vi "INITIALIZE DB CONNECTION.vi"(8 "error in (no error)":errorcluster, 9 "Password":string, 10 "User Name":string="Admin", 11 "DB PATH":path=path "E:/LabView/PPLR DATABAS.udl") -> (0 "error out":errorcluster, 3 "CONNECTED?":bool)   [LabVIEW 2024]
uses:
  <vilib>/addons/database/Connection.llb/DB Tools Open Connec (Path).vi
  <vilib>/addons/database/NI_Database_API.lvlib
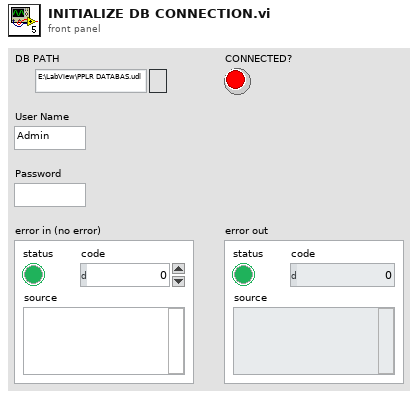
[diagram p1: front panel]
types:
  T1 = typedef "NI_Database_API.lvlib/Conn ObjectReference.ctl" = refnum<k1>
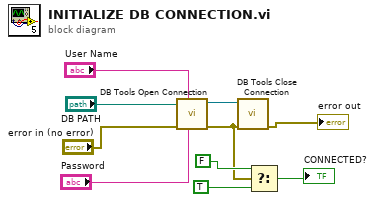
[diagram p0: block diagram]
diagram:
  n1 = call-poly <vilib>:"DB Tools Open Connection.vi"("password"="Password", "userID"="User Name", "error in (no error)"="error in (no error)", "connection information"="DB PATH") -> ("error out"=w7:errorcluster, "connection reference"=w5:T1)  [unwired: 4 in]
  n2 = call <vilib>:"DB Tools Close Connection.vi"("error in (no error)"=w7, "connection reference"=w5) -> ("error out"=→"error out":errorcluster)  [unwired: 5 in]
  n3 = Select(t=FALSE, s=w7, f=TRUE) -> (s? t:f=→"CONNECTED?":bool)
